vi "FdxCmdRxUDPBlockRead2Cvi.vi"(7 "error in (no error)":errorcluster, 8 "RxUDPBlockReadInPortArray":T1(array[cluster]) {"UDP Handle Out" format="%.0x"; "UDP Handle" format="%.0x"}, 9 "PortCountIn":u32, 10 "InstrumentHandle":u32) -> (0 "error out":errorcluster, 1 "RxUDPBlockReadIOutPortArray":T1(array[cluster]) {"UDP Handle Out" format="%.0x"; "UDP Handle" format="%.0x"}, 3 "status":i32)   [LabVIEW 2020, in "AIM664LV.lvlib"]
doc: "This function reads data from one or several UDP connection oriented ports."
uses:
  AIM664LV.lvlib
  Program Files/AIM GmbH/Arinc 664 Windows BSP 19.5.0/LabView/AFDX_LibraryAdmin.llb/FdxGlobalDllPath.vi
panel:
  # "Inputs"
  # "Outputs"
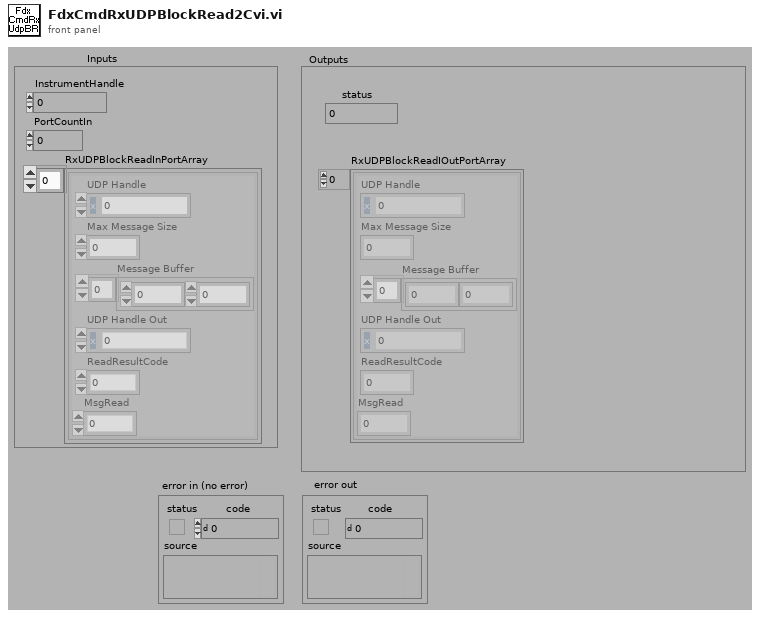
[diagram p1: front panel]
types:
  T1 = cluster{"UDP Handle":u32, "Max Message Size":u32, "Message Buffer":u8[], "UDP Handle Out":u32, "ReadResultCode":i32, "MsgRead":u32}[]
  T2 = cluster{"RxUDPBlockReadInPortArray[0]":cluster{"UDP Handle":u32, "Max Message Size":u32, "Message Buffer":u8[], "UDP Handle Out":u32, "ReadResultCode":i32, "MsgRead":u32}, "RxUDPBlockReadInPortArray[1]":cluster{"UDP Handle":u32, "Max Message Size":u32, "Message Buffer":u8[], "UDP Handle Out":u32, "ReadResultCode":i32, "MsgRead":u32}, "RxUDPBlockReadInPortArray[2]":cluster{"UDP Handle":u32, "Max Message Size":u32, "Message Buffer":u8[], "UDP Handle Out":u32, "ReadResultCode":i32, "MsgRead":u32}, "RxUDPBlockReadInPortArray[3]":cluster{"UDP Handle":u32, "Max Message Size":u32, "Message Buffer":u8[], "UDP Handle Out":u32, "ReadResultCode":i32, "MsgRead":u32}, "RxUDPBlockReadInPortArray[4]":cluster{"UDP Handle":u32, "Max Message Size":u32, "Message Buffer":u8[], "UDP Handle Out":u32, "ReadResultCode":i32, "MsgRead":u32}, "RxUDPBlockReadInPortArray[5]":cluster{"UDP Handle":u32, "Max Message Size":u32, "Message Buffer":u8[], "UDP Handle Out":u32, "ReadResultCode":i32, "MsgRead":u32}, "RxUDPBlockReadInPortArray[6]":cluster{"UDP Handle":u32, "Max Message Size":u32, "Message Buffer":u8[], "UDP Handle Out":u32, "ReadResultCode":i32, "MsgRead":u32}, "RxUDPBlockReadInPortArray[7]":cluster{"UDP Handle":u32, "Max Message Size":u32, "Message Buffer":u8[], "UDP Handle Out":u32, "ReadResultCode":i32, "MsgRead":u32}, "RxUDPBlockReadInPortArray[8]":cluster{"UDP Handle":u32, "Max Message Size":u32, "Message Buffer":u8[], "UDP Handle Out":u32, "ReadResultCode":i32, "MsgRead":u32}, "RxUDPBlockReadInPortArray[9]":cluster{"UDP Handle":u32, "Max Message Size":u32, "Message Buffer":u8[], "UDP Handle Out":u32, "ReadResultCode":i32, "MsgRead":u32}, "RxUDPBlockReadInPortArray[10]":cluster{"UDP Handle":u32, "Max Message Size":u32, "Message Buffer":u8[], "UDP Handle Out":u32, "ReadResultCode":i32, "MsgRead":u32}, "RxUDPBlockReadInPortArray[11]":cluster{"UDP Handle":u32, "Max Message Size":u32, "Message Buffer":u8[], "UDP Handle Out":u32, "ReadResultCode":i32, "MsgRead":u32}, "RxUDPBlockReadInPortArray[12]":cluster{"UDP Handle":u32, "Max Message Size":u32, "Message Buffer":u8[], "UDP Handle Out":u32, "ReadResultCode":i32, "MsgRead":u32}, "RxUDPBlockReadInPortArray[13]":cluster{"UDP Handle":u32, "Max Message Size":u32, "Message Buffer":u8[], "UDP Handle Out":u32, "ReadResultCode":i32, "MsgRead":u32}, "RxUDPBlockReadInPortArray[14]":cluster{"UDP Handle":u32, "Max Message Size":u32, "Message Buffer":u8[], "UDP Handle Out":u32, "ReadResultCode":i32, "MsgRead":u32}, "RxUDPBlockReadInPortArray[15]":cluster{"UDP Handle":u32, "Max Message Size":u32, "Message Buffer":u8[], "UDP Handle Out":u32, "ReadResultCode":i32, "MsgRead":u32}, "RxUDPBlockReadInPortArray[16]":cluster{"UDP Handle":u32, "Max Message Size":u32, "Message Buffer":u8[], "UDP Handle Out":u32, "ReadResultCode":i32, "MsgRead":u32}, "RxUDPBlockReadInPortArray[17]":cluster{"UDP Handle":u32, "Max Message Size":u32, "Message Buffer":u8[], "UDP Handle Out":u32, "ReadResultCode":i32, "MsgRead":u32}, "RxUDPBlockReadInPortArray[18]":cluster{"UDP Handle":u32, "Max Message Size":u32, "Message Buffer":u8[], "UDP Handle Out":u32, "ReadResultCode":i32, "MsgRead":u32}, "RxUDPBlockReadInPortArray[19]":cluster{"UDP Handle":u32, "Max Message Size":u32, "Message Buffer":u8[], "UDP Handle Out":u32, "ReadResultCode":i32, "MsgRead":u32}, "RxUDPBlockReadInPortArray[20]":cluster{"UDP Handle":u32, "Max Message Size":u32, "Message Buffer":u8[], "UDP Handle Out":u32, "ReadResultCode":i32, "MsgRead":u32}, "RxUDPBlockReadInPortArray[21]":cluster{"UDP Handle":u32, "Max Message Size":u32, "Message Buffer":u8[], "UDP Handle Out":u32, "ReadResultCode":i32, "MsgRead":u32}, "RxUDPBlockReadInPortArray[22]":cluster{"UDP Handle":u32, "Max Message Size":u32, "Message Buffer":u8[], "UDP Handle Out":u32, "ReadResultCode":i32, "MsgRead":u32}, "RxUDPBlockReadInPortArray[23]":cluster{"UDP Handle":u32, "Max Message Size":u32, "Message Buffer":u8[], "UDP Handle Out":u32, "ReadResultCode":i32, "MsgRead":u32}, "RxUDPBlockReadInPortArray[24]":cluster{"UDP Handle":u32, "Max Message Size":u32, "Message Buffer":u8[], "UDP Handle Out":u32, "ReadResultCode":i32, "MsgRead":u32}, "RxUDPBlockReadInPortArray[25]":cluster{"UDP Handle":u32, "Max Message Size":u32, "Message Buffer":u8[], "UDP Handle Out":u32, "ReadResultCode":i32, "MsgRead":u32}, "RxUDPBlockReadInPortArray[26]":cluster{"UDP Handle":u32, "Max Message Size":u32, "Message Buffer":u8[], "UDP Handle Out":u32, "ReadResultCode":i32, "MsgRead":u32}, "RxUDPBlockReadInPortArray[27]":cluster{"UDP Handle":u32, "Max Message Size":u32, "Message Buffer":u8[], "UDP Handle Out":u32, "ReadResultCode":i32, "MsgRead":u32}, "RxUDPBlockReadInPortArray[28]":cluster{"UDP Handle":u32, "Max Message Size":u32, "Message Buffer":u8[], "UDP Handle Out":u32, "ReadResultCode":i32, "MsgRead":u32}, "RxUDPBlockReadInPortArray[29]":cluster{"UDP Handle":u32, "Max Message Size":u32, "Message Buffer":u8[], "UDP Handle Out":u32, "ReadResultCode":i32, "MsgRead":u32}, "RxUDPBlockReadInPortArray[30]":cluster{"UDP Handle":u32, "Max Message Size":u32, "Message Buffer":u8[], "UDP Handle Out":u32, "ReadResultCode":i32, "MsgRead":u32}, "RxUDPBlockReadInPortArray[31]":cluster{"UDP Handle":u32, "Max Message Size":u32, "Message Buffer":u8[], "UDP Handle Out":u32, "ReadResultCode":i32, "MsgRead":u32}, "RxUDPBlockReadInPortArray[32]":cluster{"UDP Handle":u32, "Max Message Size":u32, "Message Buffer":u8[], "UDP Handle Out":u32, "ReadResultCode":i32, "MsgRead":u32}, "RxUDPBlockReadInPortArray[33]":cluster{"UDP Handle":u32, "Max Message Size":u32, "Message Buffer":u8[], "UDP Handle Out":u32, "ReadResultCode":i32, "MsgRead":u32}, "RxUDPBlockReadInPortArray[34]":cluster{"UDP Handle":u32, "Max Message Size":u32, "Message Buffer":u8[], "UDP Handle Out":u32, "ReadResultCode":i32, "MsgRead":u32}, "RxUDPBlockReadInPortArray[35]":cluster{"UDP Handle":u32, "Max Message Size":u32, "Message Buffer":u8[], "UDP Handle Out":u32, "ReadResultCode":i32, "MsgRead":u32}, "RxUDPBlockReadInPortArray[36]":cluster{"UDP Handle":u32, "Max Message Size":u32, "Message Buffer":u8[], "UDP Handle Out":u32, "ReadResultCode":i32, "MsgRead":u32}, "RxUDPBlockReadInPortArray[37]":cluster{"UDP Handle":u32, "Max Message Size":u32, "Message Buffer":u8[], "UDP Handle Out":u32, "ReadResultCode":i32, "MsgRead":u32}, "RxUDPBlockReadInPortArray[38]":cluster{"UDP Handle":u32, "Max Message Size":u32, "Message Buffer":u8[], "UDP Handle Out":u32, "ReadResultCode":i32, "MsgRead":u32}, "RxUDPBlockReadInPortArray[39]":cluster{"UDP Handle":u32, "Max Message Size":u32, "Message Buffer":u8[], "UDP Handle Out":u32, "ReadResultCode":i32, "MsgRead":u32}, "RxUDPBlockReadInPortArray[40]":cluster{"UDP Handle":u32, "Max Message Size":u32, "Message Buffer":u8[], "UDP Handle Out":u32, "ReadResultCode":i32, "MsgRead":u32}, "RxUDPBlockReadInPortArray[41]":cluster{"UDP Handle":u32, "Max Message Size":u32, "Message Buffer":u8[], "UDP Handle Out":u32, "ReadResultCode":i32, "MsgRead":u32}, "RxUDPBlockReadInPortArray[42]":cluster{"UDP Handle":u32, "Max Message Size":u32, "Message Buffer":u8[], "UDP Handle Out":u32, "ReadResultCode":i32, "MsgRead":u32}, "RxUDPBlockReadInPortArray[43]":cluster{"UDP Handle":u32, "Max Message Size":u32, "Message Buffer":u8[], "UDP Handle Out":u32, "ReadResultCode":i32, "MsgRead":u32}, "RxUDPBlockReadInPortArray[44]":cluster{"UDP Handle":u32, "Max Message Size":u32, "Message Buffer":u8[], "UDP Handle Out":u32, "ReadResultCode":i32, "MsgRead":u32}, "RxUDPBlockReadInPortArray[45]":cluster{"UDP Handle":u32, "Max Message Size":u32, "Message Buffer":u8[], "UDP Handle Out":u32, "ReadResultCode":i32, "MsgRead":u32}, "RxUDPBlockReadInPortArray[46]":cluster{"UDP Handle":u32, "Max Message Size":u32, "Message Buffer":u8[], "UDP Handle Out":u32, "ReadResultCode":i32, "MsgRead":u32}, "RxUDPBlockReadInPortArray[47]":cluster{"UDP Handle":u32, "Max Message Size":u32, "Message Buffer":u8[], "UDP Handle Out":u32, "ReadResultCode":i32, "MsgRead":u32}, "RxUDPBlockReadInPortArray[48]":cluster{"UDP Handle":u32, "Max Message Size":u32, "Message Buffer":u8[], "UDP Handle Out":u32, "ReadResultCode":i32, "MsgRead":u32}, "RxUDPBlockReadInPortArray[49]":cluster{"UDP Handle":u32, "Max Message Size":u32, "Message Buffer":u8[], "UDP Handle Out":u32, "ReadResultCode":i32, "MsgRead":u32}, "RxUDPBlockReadInPortArray[50]":cluster{"UDP Handle":u32, "Max Message Size":u32, "Message Buffer":u8[], "UDP Handle Out":u32, "ReadResultCode":i32, "MsgRead":u32}, "RxUDPBlockReadInPortArray[51]":cluster{"UDP Handle":u32, "Max Message Size":u32, "Message Buffer":u8[], "UDP Handle Out":u32, "ReadResultCode":i32, "MsgRead":u32}, "RxUDPBlockReadInPortArray[52]":cluster{"UDP Handle":u32, "Max Message Size":u32, "Message Buffer":u8[], "UDP Handle Out":u32, "ReadResultCode":i32, "MsgRead":u32}, "RxUDPBlockReadInPortArray[53]":cluster{"UDP Handle":u32, "Max Message Size":u32, "Message Buffer":u8[], "UDP Handle Out":u32, "ReadResultCode":i32, "MsgRead":u32}, "RxUDPBlockReadInPortArray[54]":cluster{"UDP Handle":u32, "Max Message Size":u32, "Message Buffer":u8[], "UDP Handle Out":u32, "ReadResultCode":i32, "MsgRead":u32}, "RxUDPBlockReadInPortArray[55]":cluster{"UDP Handle":u32, "Max Message Size":u32, "Message Buffer":u8[], "UDP Handle Out":u32, "ReadResultCode":i32, "MsgRead":u32}, "RxUDPBlockReadInPortArray[56]":cluster{"UDP Handle":u32, "Max Message Size":u32, "Message Buffer":u8[], "UDP Handle Out":u32, "ReadResultCode":i32, "MsgRead":u32}, "RxUDPBlockReadInPortArray[57]":cluster{"UDP Handle":u32, "Max Message Size":u32, "Message Buffer":u8[], "UDP Handle Out":u32, "ReadResultCode":i32, "MsgRead":u32}, "RxUDPBlockReadInPortArray[58]":cluster{"UDP Handle":u32, "Max Message Size":u32, "Message Buffer":u8[], "UDP Handle Out":u32, "ReadResultCode":i32, "MsgRead":u32}, "RxUDPBlockReadInPortArray[59]":cluster{"UDP Handle":u32, "Max Message Size":u32, "Message Buffer":u8[], "UDP Handle Out":u32, "ReadResultCode":i32, "MsgRead":u32}, "RxUDPBlockReadInPortArray[60]":cluster{"UDP Handle":u32, "Max Message Size":u32, "Message Buffer":u8[], "UDP Handle Out":u32, "ReadResultCode":i32, "MsgRead":u32}, "RxUDPBlockReadInPortArray[61]":cluster{"UDP Handle":u32, "Max Message Size":u32, "Message Buffer":u8[], "UDP Handle Out":u32, "ReadResultCode":i32, "MsgRead":u32}, "RxUDPBlockReadInPortArray[62]":cluster{"UDP Handle":u32, "Max Message Size":u32, "Message Buffer":u8[], "UDP Handle Out":u32, "ReadResultCode":i32, "MsgRead":u32}, "RxUDPBlockReadInPortArray[63]":cluster{"UDP Handle":u32, "Max Message Size":u32, "Message Buffer":u8[], "UDP Handle Out":u32, "ReadResultCode":i32, "MsgRead":u32}, "RxUDPBlockReadInPortArray[64]":cluster{"UDP Handle":u32, "Max Message Size":u32, "Message Buffer":u8[], "UDP Handle Out":u32, "ReadResultCode":i32, "MsgRead":u32}, "RxUDPBlockReadInPortArray[65]":cluster{"UDP Handle":u32, "Max Message Size":u32, "Message Buffer":u8[], "UDP Handle Out":u32, "ReadResultCode":i32, "MsgRead":u32}, "RxUDPBlockReadInPortArray[66]":cluster{"UDP Handle":u32, "Max Message Size":u32, "Message Buffer":u8[], "UDP Handle Out":u32, "ReadResultCode":i32, "MsgRead":u32}, "RxUDPBlockReadInPortArray[67]":cluster{"UDP Handle":u32, "Max Message Size":u32, "Message Buffer":u8[], "UDP Handle Out":u32, "ReadResultCode":i32, "MsgRead":u32}, "RxUDPBlockReadInPortArray[68]":cluster{"UDP Handle":u32, "Max Message Size":u32, "Message Buffer":u8[], "UDP Handle Out":u32, "ReadResultCode":i32, "MsgRead":u32}, "RxUDPBlockReadInPortArray[69]":cluster{"UDP Handle":u32, "Max Message Size":u32, "Message Buffer":u8[], "UDP Handle Out":u32, "ReadResultCode":i32, "MsgRead":u32}, "RxUDPBlockReadInPortArray[70]":cluster{"UDP Handle":u32, "Max Message Size":u32, "Message Buffer":u8[], "UDP Handle Out":u32, "ReadResultCode":i32, "MsgRead":u32}, "RxUDPBlockReadInPortArray[71]":cluster{"UDP Handle":u32, "Max Message Size":u32, "Message Buffer":u8[], "UDP Handle Out":u32, "ReadResultCode":i32, "MsgRead":u32}, "RxUDPBlockReadInPortArray[72]":cluster{"UDP Handle":u32, "Max Message Size":u32, "Message Buffer":u8[], "UDP Handle Out":u32, "ReadResultCode":i32, "MsgRead":u32}, "RxUDPBlockReadInPortArray[73]":cluster{"UDP Handle":u32, "Max Message Size":u32, "Message Buffer":u8[], "UDP Handle Out":u32, "ReadResultCode":i32, "MsgRead":u32}, ...}
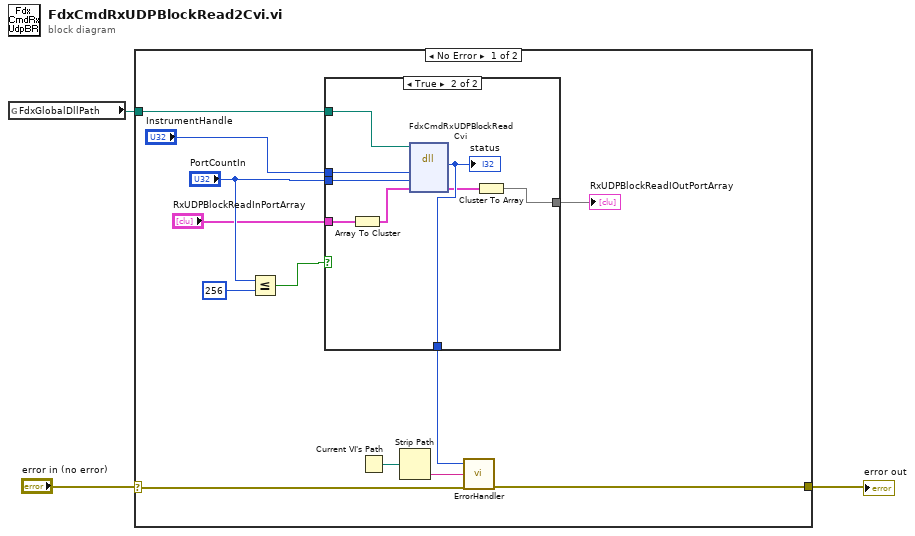
[diagram p0: block diagram]
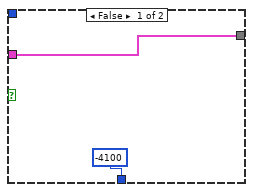
[diagram p2: hidden frame]
diagram:
  n1 = global read "FdxGlobalDllPath.vi" "FdxGlobalDllPath"() -> (w1:path)
  n2 = case shown="No Error" "error in (no error)" {
    selector: "error in (no error)" -> [w11 w26]
    tunnel: [w15 w26] -> w3
    tunnel: w1 -> [w9 _]
    frame No Error {
      n3 = Less Or Equal?(x="PortCountIn", y=u32 256) -> (x <= y?=w5:bool)
      n4 = case shown="True" w5 {
        tunnel: [-4100 ("status") w25] -> w14
        tunnel: "InstrumentHandle" -> [_ w24]
        tunnel: w9 -> [_ w23]
        tunnel: [w17 w21] -> w8
        tunnel: "PortCountIn" -> [_ w20]
        tunnel: "RxUDPBlockReadInPortArray" -> [w17 w19]
        frame False {
        }
        frame True {
          n5 = Array To Cluster(array=w19) -> (cluster=w18:T2)
          n6 = dll-call lib="aim_fdx.19.dll" fn="FdxCmdRxUDPBlockReadCvi"(path in=w23, "InstrumentHandle"=w24, "PortCountIn"=w20, "UdpBlockReadInPortArray"=w18) -> ("status"=w25:i32, "UdpBlockReadInPortArray"=w22:T2)  [unwired: 4 in, 2 out]
          "status" <- w25
          n7 = Cluster To Array(cluster=w22) -> (array=w21:T1)
        }
      }
      "RxUDPBlockReadIOutPortArray" <- w8
      n8 = Current VI's Path() -> (path=w12:path)
      n9 = Strip Path(path=w12) -> (name=w10:string)  [unwired: 1 out]
      n10 = call "ErrorHandler.vi"("error in (no error)"=w11, "String"=w10, "Numeric"=w14) -> ("error out"=w15:errorcluster)
    }
    frame Error {
    }
  }
  "error out" <- w3
